vi "Read CFG File.vi"(8 "error in (no error)":errorcluster, 10 "File path":path, 11 "Common Measurements Interface in":refnum<class "Common Measurements Interface.lvclass">) -> (0 "error out":errorcluster, 2 "Section":string, 3 "Common Measurements Interface out":refnum<class "Common Measurements Interface.lvclass">)   [LabVIEW 2015, in "Common Measurements Interface.lvclass"]
uses:
  Common Measurements Interface.lvclass
  Common Measurements Interface.lvclass/Common Measurements Interface.ctl
  Queued Listbox/Queued Listbox.xctl
  Read Measurements Menu.vi
  Mag Lab Measure Interface/Interface with menu/Interface with menu.lvclass
  <vilib>/Utility/config.llb/NI_LVConfig.lvlib
  Mag Lab Error Handler/Mag Lab Error Handler.lvclass
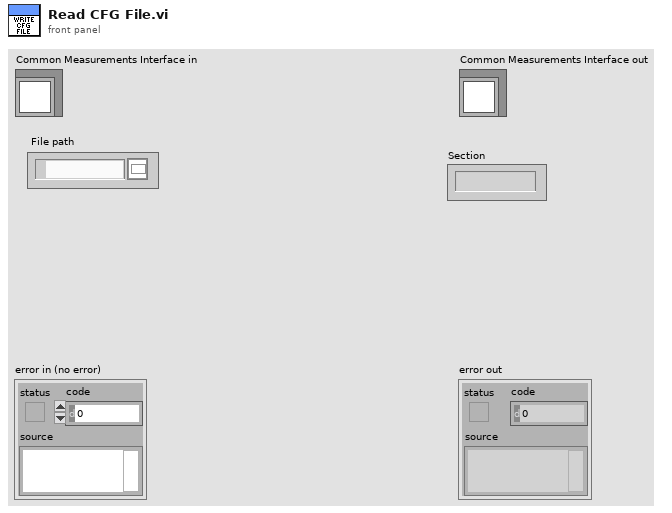
[diagram p1: front panel]
types:
  T1 = typedef "NI_LVConfig.lvlib/Config Data RefNum.ctl" = refnum<k1>
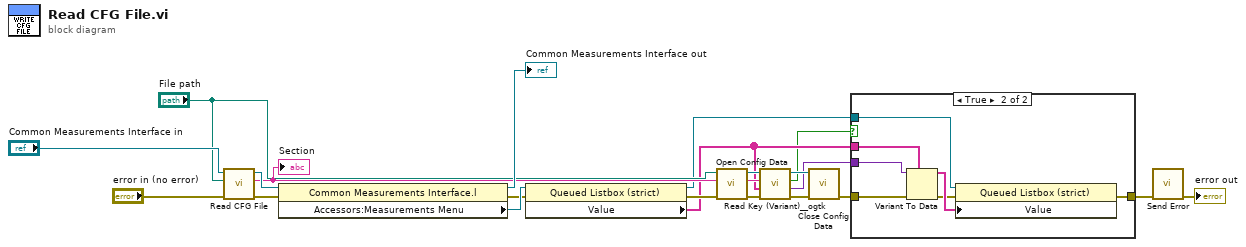
[diagram p0: block diagram]
diagram:
  n1 = call-parent "Read CFG File.vi"("error in (no error)"="error in (no error)", "File path"="File path", "Mag Lab Root in"="Common Measurements Interface in") -> ("error out"=w15:errorcluster, "Section"=w11:string, "Mag Lab Root out"=w21:refnum<class "Common Measurements Interface.lvclass">)  [unwired: 6 in]
  "Section" <- w11
  n2 = property class="Common Measurements Interface.l"(reference=w21, error in=w15) -> (reference out=→"Common Measurements Interface out":refnum<class "Common Measurements Interface.lvclass">, error out=w16:errorcluster, "Accessors:Measurements Menu"=w17:refnum<vi>)
  n3 = property class="Queued Listbox (strict)"(reference=w17, error in=w16) -> (reference out=w5:refnum<vi>, error out=w13:errorcluster, "Value"=w3:string[])
  n4 = call <vilib>:"Open Config Data.vi"("error in (no error)"=w13, "configuration file path"="File path") -> ("error out"=w10:errorcluster, "refnum"=w12:T1)  [unwired: 7 in, 1 out]
  n5 = call <userlib>:"Read Key (Variant)__ogtk.vi"("section"=w11, "error in (no error)"=w10, "type"=w3, "refnum"=w12) -> ("error out"=w9:errorcluster, "key-value"=w4:variant, "found?"=w1:bool, "refnum out"=w8:T1)  [unwired: 4 in]
  n6 = call <vilib>:"Close Config Data.vi"("error in (no error)"=w9, "refnum"=w8) -> ("error out"=w2:errorcluster)  [unwired: 8 in, 1 out]
  n7 = case shown="True" w1 {
    tunnel: [w22 w29] -> w6
    tunnel: w5 -> [_ w28]
    tunnel: w4 -> [_ w27]
    tunnel: w3 -> [_ w26]
    tunnel: w2 -> [w22 w23]
    frame False {
    }
    frame True {
      n8 = Variant To Data(error in=w23, type=w26, Variant=w27) -> (data=w25:string[], error out=w24:errorcluster)
      n9 = property class="Queued Listbox (strict)"(reference=w28, error in=w24, "Value"=w25) -> (error out=w29:errorcluster)  [unwired: 1 out]
    }
  }
  n10 = call "Send Error.vi"("error in (no error)"=w6) -> ("error out"=→"error out":errorcluster)  [unwired: 9 in, 1 out]
